vi "AWS-S3-GetObjectData.vi"(0 "AWS-S3-API":refnum<class "AWS-S3-API.lvclass">, 5 "Object Key":string, 7 "Object Bucket":string, 9 "Object VersionID":string, 11 "error in":errorcluster) -> (4 "AWS-S3-API out":refnum<class "AWS-S3-API.lvclass">, 6 "Object Data":string, 15 "error out":errorcluster)   [LabVIEW 2012, in "AWS-S3-API.lvclass"]
uses:
  AWS-S3-API.lvclass
  C:/Users/Jack/repo/visualize/Dependencies/aws/AWS-SDK/AWSSDK.dll
  AWS-SDK/AWSSDK.dll
panel:
  # "Inputs"
  # "Outputs"
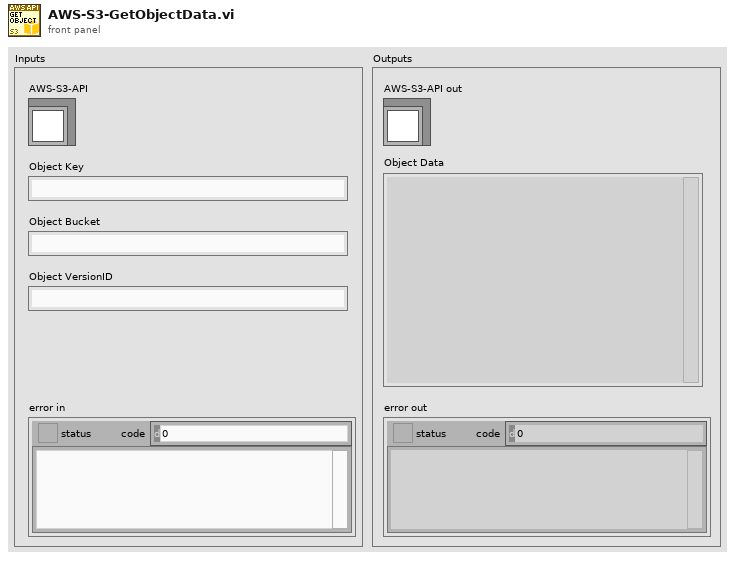
[diagram p1: front panel]
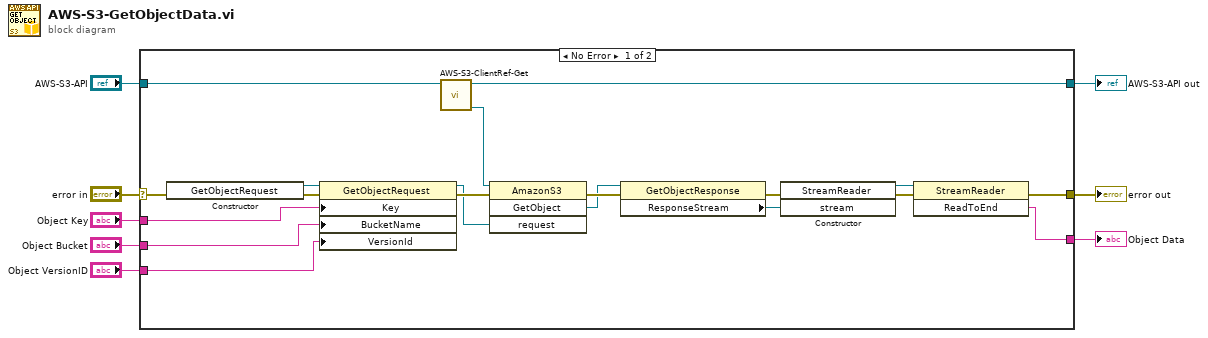
[diagram p0: block diagram]
diagram:
  n1 = case shown="No Error" "error in" {
    selector: "error in" -> [w23 w29]
    tunnel: [w21 w29] -> w8
    tunnel: [w9 w28] -> w6
    tunnel: "AWS-S3-API" -> [w10 w28]
    tunnel: "Object Key" -> [w15 _]
    tunnel: "Object Bucket" -> [w16 _]
    tunnel: "Object VersionID" -> [w24 _]
    tunnel: [w14 _] -> w1
    frame No Error {
      n2 = constructor class="GetObjectRequest"(error in=w23) -> (reference out=w25:refnum<k24>, error out=w27:errorcluster)  [unwired: 2 in, 1 out]
      n3 = property class="GetObjectRequest"(reference=w25, error in=w27, "Key"=w15, "BucketName"=w16, "VersionId"=w24) -> (reference out=w22:refnum<k24>, error out=w26:errorcluster)
      n4 = call "AWS-S3-ClientRef-Get.vi"("AWS-S3-API"=w10) -> ("S3 Client ref"=w11:refnum<k24>, "AWS-S3-API out"=w9:refnum<class "AWS-S3-API.lvclass">)  [unwired: 9 in]
      n5 = invoke class="AmazonS3" method="GetObject"(reference=w11, error in=w26, "request"=w22) -> (error out=w20:errorcluster, "GetObject"=w19:refnum<k24>)  [unwired: 1 in, 2 out]
      n6 = property class="GetObjectResponse"(reference=w19, error in=w20) -> (error out=w13:errorcluster, "ResponseStream"=w18:refnum<k24>)  [unwired: 1 out]
      n7 = constructor class="StreamReader"(error in=w13, "stream"=w18) -> (reference out=w17:refnum<k24>, error out=w12:errorcluster)  [unwired: 2 in, 2 out]
      n8 = invoke class="StreamReader" method="ReadToEnd"(reference=w17, error in=w12) -> (error out=w21:errorcluster, "ReadToEnd"=w14:string)  [unwired: 1 in, 1 out]
    }
    frame Error {
    }
  }
  "error out" <- w8
  "AWS-S3-API out" <- w6
  "Object Data" <- w1
